vi "To 2D Path Tree Data.vi"(10 "2D Path":path[][](array[path])) -> (3 "2D Path Tree Data":refnum<class "2D Path.lvclass">)   [LabVIEW 2020, in "NI_VIAnCFGDataStructure.lvlib" / "2D Path.lvclass"]
doc: "Convert a 2D Path value to Tree Data type."
uses:
  <vilib>/addons/analyzer/VIAnCFGDataStructure/Data Types/2D Path/2D Path.lvclass
  <vilib>/addons/analyzer/VIAnCFGDataStructure/Data Types/2D Path/2D Path.lvclass/2D Path.ctl
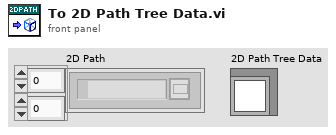
[diagram p1: front panel]
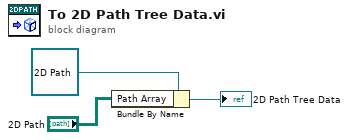
[diagram p0: block diagram]
diagram:
  n1 = Bundle By Name(cluster=refnum<class "2D Path.lvclass"> refnum ("Tree API.lvlib:2D Path.lvclass"), "Path Array"="2D Path") -> (→"2D Path Tree Data":refnum<class "2D Path.lvclass">)
